vi "Teleop Cmd Changed.vi"(8 "Epsilon":dbl, 10 "New Teleop Values":T1, 11 "Prev Teleop Values":T1) -> (3 "Boolean":bool)   [LabVIEW 2014]
uses:
  TeleopCmd.ctl
  CmdFlag.ctl
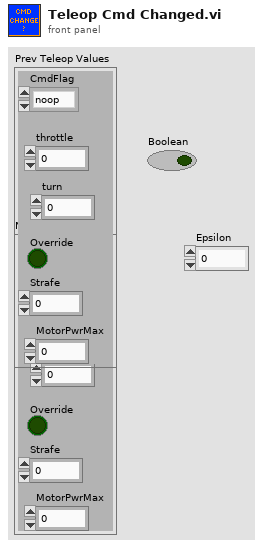
[diagram p1: front panel]
types:
  T1 = typedef "TeleopCmd.ctl" = cluster{"CmdFlag":T2, "throttle":dbl, "turn":dbl, "Override":bool, "Strafe":dbl, "MotorPwrMax":dbl}
  T2 = typedef "CmdFlag.ctl" = enum16{"noop", "suspend", "resume"}
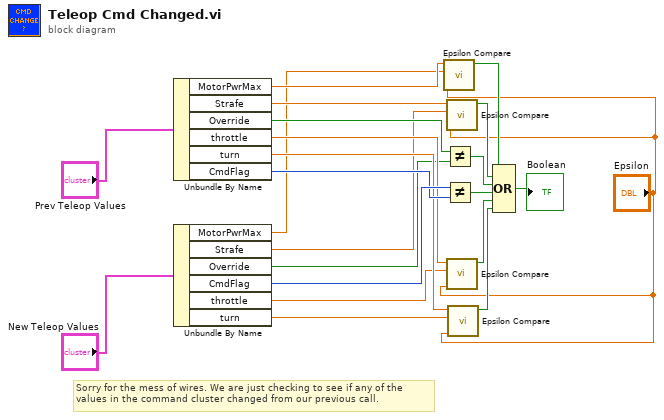
[diagram p0: block diagram]
diagram:
  # "Sorry for the mess of wires. We are just checking to see if any of the \nvalues in the command cluster changed from our previous call."
  n1 = Unbundle By Name("Prev Teleop Values") -> ("MotorPwrMax"=w4:dbl, "Strafe"=w7:dbl, "Override"=w10:bool, "throttle"=w16:dbl, "turn"=w15:dbl, "CmdFlag"=w17:T2)
  n2 = Unbundle By Name("New Teleop Values") -> ("MotorPwrMax"=w3:dbl, "Strafe"=w6:dbl, "Override"=w9:bool, "CmdFlag"=w19:T2, "throttle"=w14:dbl, "turn"=w13:dbl)
  n3 = call "Epsilon Compare.vi"("Epsilon"="Epsilon", "Value2"=w3, "Value1"=w4) -> ("Boolean"=w2:bool)  [unwired: 8 in]
  n4 = Not Equal?(x=w10, y=w9) -> (x != y?=w8:bool)
  n5 = Not Equal?(x=w19, y=w17) -> (x != y?=w18:bool)
  n6 = call "Epsilon Compare.vi"("Epsilon"="Epsilon", "Value2"=w6, "Value1"=w7) -> ("Boolean"=w5:bool)  [unwired: 8 in]
  n7 = call "Epsilon Compare.vi"("Epsilon"="Epsilon", "Value2"=w14, "Value1"=w16) -> ("Boolean"=w12:bool)  [unwired: 8 in]
  n8 = call "Epsilon Compare.vi"("Epsilon"="Epsilon", "Value2"=w13, "Value1"=w15) -> ("Boolean"=w11:bool)  [unwired: 8 in]
  n9 = Compound Arithmetic op=OR(w2, w5, w8, w18, w12, w11) -> (→"Boolean":bool)
